vi "Calculate Measurement Timeout.vi"(2 "overhead":dbl[unit]=0.25, 3 "number of samples":i32=1, 4 "sample rate":dbl[unit]=nan) -> (0 "elapsed time":dbl[unit]=nan format="%_3g", 1 "timeout":dbl[unit]=nan format="%_3g")   [LabVIEW 2010]
doc: "Calculates the expected measurement time (elapsed time) based on the product of the sample rate and number of samples. Calculates the required timeout based on the elapsed time plus an overhead time interval."
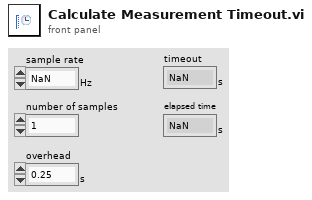
[diagram p1: front panel]
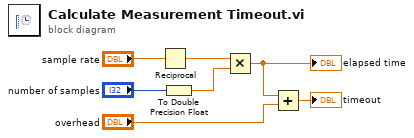
[diagram p0: block diagram]
diagram:
  n1 = Reciprocal(x="sample rate") -> (1/x=w4:dbl[unit])
  n2 = To Double Precision Float(number="number of samples") -> (double precision float=w6:dbl)
  n3 = Multiply(x=w4, y=w6) -> (x*y=w1:dbl[unit])
  "elapsed time" <- w1
  n4 = Add(x=w1, y="overhead") -> (x+y=→"timeout":dbl[unit])
